vi "Fetch Backlog (U32).vi"(8 "error in":errorcluster, 11 "FPGA Session":T1) -> (0 "error out":errorcluster, 1 "Fetch Backlog":u32, 3 "FPGA Session":T1)   [LabVIEW 2011, in "FlexRIO Host Library (User).lvlib"]
uses:
  <userlib>/FlexRIO Host Library/FlexRIO Host Library (User).lvlib
  <vilib>/rvi/interface/nirviMethod/nirviMethod.xnode
  <userlib>/FlexRIO Host Library/FlexRIO Host API/Session/FPGA Session Ref.ctl
  OCT Reference Design/FPGA Bitfiles/OCTDigitizer_FPGABoard_AcquireDatawithout DRAM.lvbitx
  <vilib>/FPGAPlugInAG/PXIe-7965R/niLvFpga_ReadFifo_PXIe-7965R.vi
  <vilib>/rvi/errors/niLvFpgaMergeErrorWithErrorCode.vi
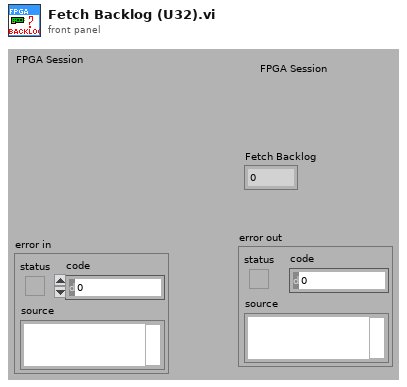
[diagram p1: front panel]
types:
  T1 = typedef "FlexRIO Host Library (User).lvlib/FPGA Session Ref.ctl" = refnum<k20>
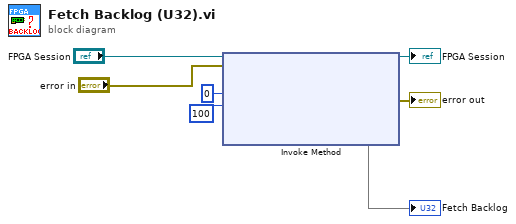
[diagram p0: block diagram]
diagram:
  n1 = xnode "Invoke Method"("FPGA VI Reference In"="FPGA Session", "error in"="error in", "Number of Elements"=u32 0, "Timeout (ms)"=100) -> ("FPGA VI Reference Out"=→"FPGA Session":T1, "error out"=→"error out":errorcluster, "Elements Remaining"=→"Fetch Backlog")  [unwired: 1 out]
